vi "Main_Equip_1kw_ref742.vi"() -> ()   [LabVIEW 2025]
panel:
  out "hardware name":string
  out "isOnline 2":bool
  out "IndexSup":i32
  out "IndexInf":i32
  in  "Verifica":bool
  out "High Time":sgl format="%#_3g"
  out "Low Time":sgl format="%#_3g"
  in  "High Temp.":sgl
  in  "Low Temp.":sgl
  out "Temps":sgl caption="Time" format="%.1f"
  out "Calibration result:":bool
  out "error out_USB":errorcluster
  out "Nom Sensor Temperatura":string
  in  "Dades":sgl[](array[numeric])
  in  "Guardar 24h":bool caption="Informe"
  out "Dies":u8 caption="NumDies"
  in  "Reset_AutoSave 24":bool
  in  "mT1":sgl caption="Temperatura_1" format="%.1f"
  out "Maxim":sgl
  in  "BtSalir":bool caption="Sortir"
  in  "Reset_AutoSave":bool
  in  "Test name:":string
  out "Gràfiques T-Temps":cluster{"Value":sgl[], "Value":sgl[]}[](graph)
  in  "Datos OK":bool
  out "DadesComplertes":sgl[](array[numeric])
  in  "Grafica_OK":bool=TRUE
  out "Tabla":sgl[][](array[numeric])
  in  "Registro OK":bool=TRUE
  in  "time out":bool
  in  "Reset_gráfica":bool
  in  "Reset_Time":bool
  in  "Tiempo_string":string[](array[string])
  out "Elapsed Time (s)":i32
  out "Ensayo activo":bool
  out "FSenseTara":sgl caption="Fuerza - N"
  in  "CaptadorF":u16(ring) caption="Unidades" items=["25kg"=5]
  in  "PendentLlum":sgl caption="Força" format="%.1f"
  out "FactorsUnitatsPendents_F":dbl[](array[numeric])
  out "ConversioUnitatsF":dbl[](array[numeric])=[1.0, 9.8756, 2.2]
  out "ArraiUnitats":cluster{"String":string, "Value":u16}[](array[cluster])=[{"String"="kg", "Value"=0}, {"String"="N", "Value"=1}, {"String"="g", "Value"=2}, {"String"="daN", "Value"=3}, {"String"="cN", "Value"=4}, {"String"="KN", "Value"=5}, {"String"="lb", "Value"=6}]
  out "Tara":sgl caption="Força" format="%.1f"
  out "Temperatura1":sgl caption="Temperature" format="%.1f"
  out "PendentsT":sgl[](array[numeric])
  in  "Salir":bool caption="Sortir"
  in  "Ensayonuevo":bool caption="New Test"
  in  "Guardar":bool
  in  "Iniciar / Finalizar":bool=TRUE caption="Finalitzar prova"
  in  "UnidadesF":u16(ring) caption="Unidades" items=["kg", "N", "g"]
  in  "BtTaraPot":bool caption="TARA"
  # "sg"
  # "ºC"
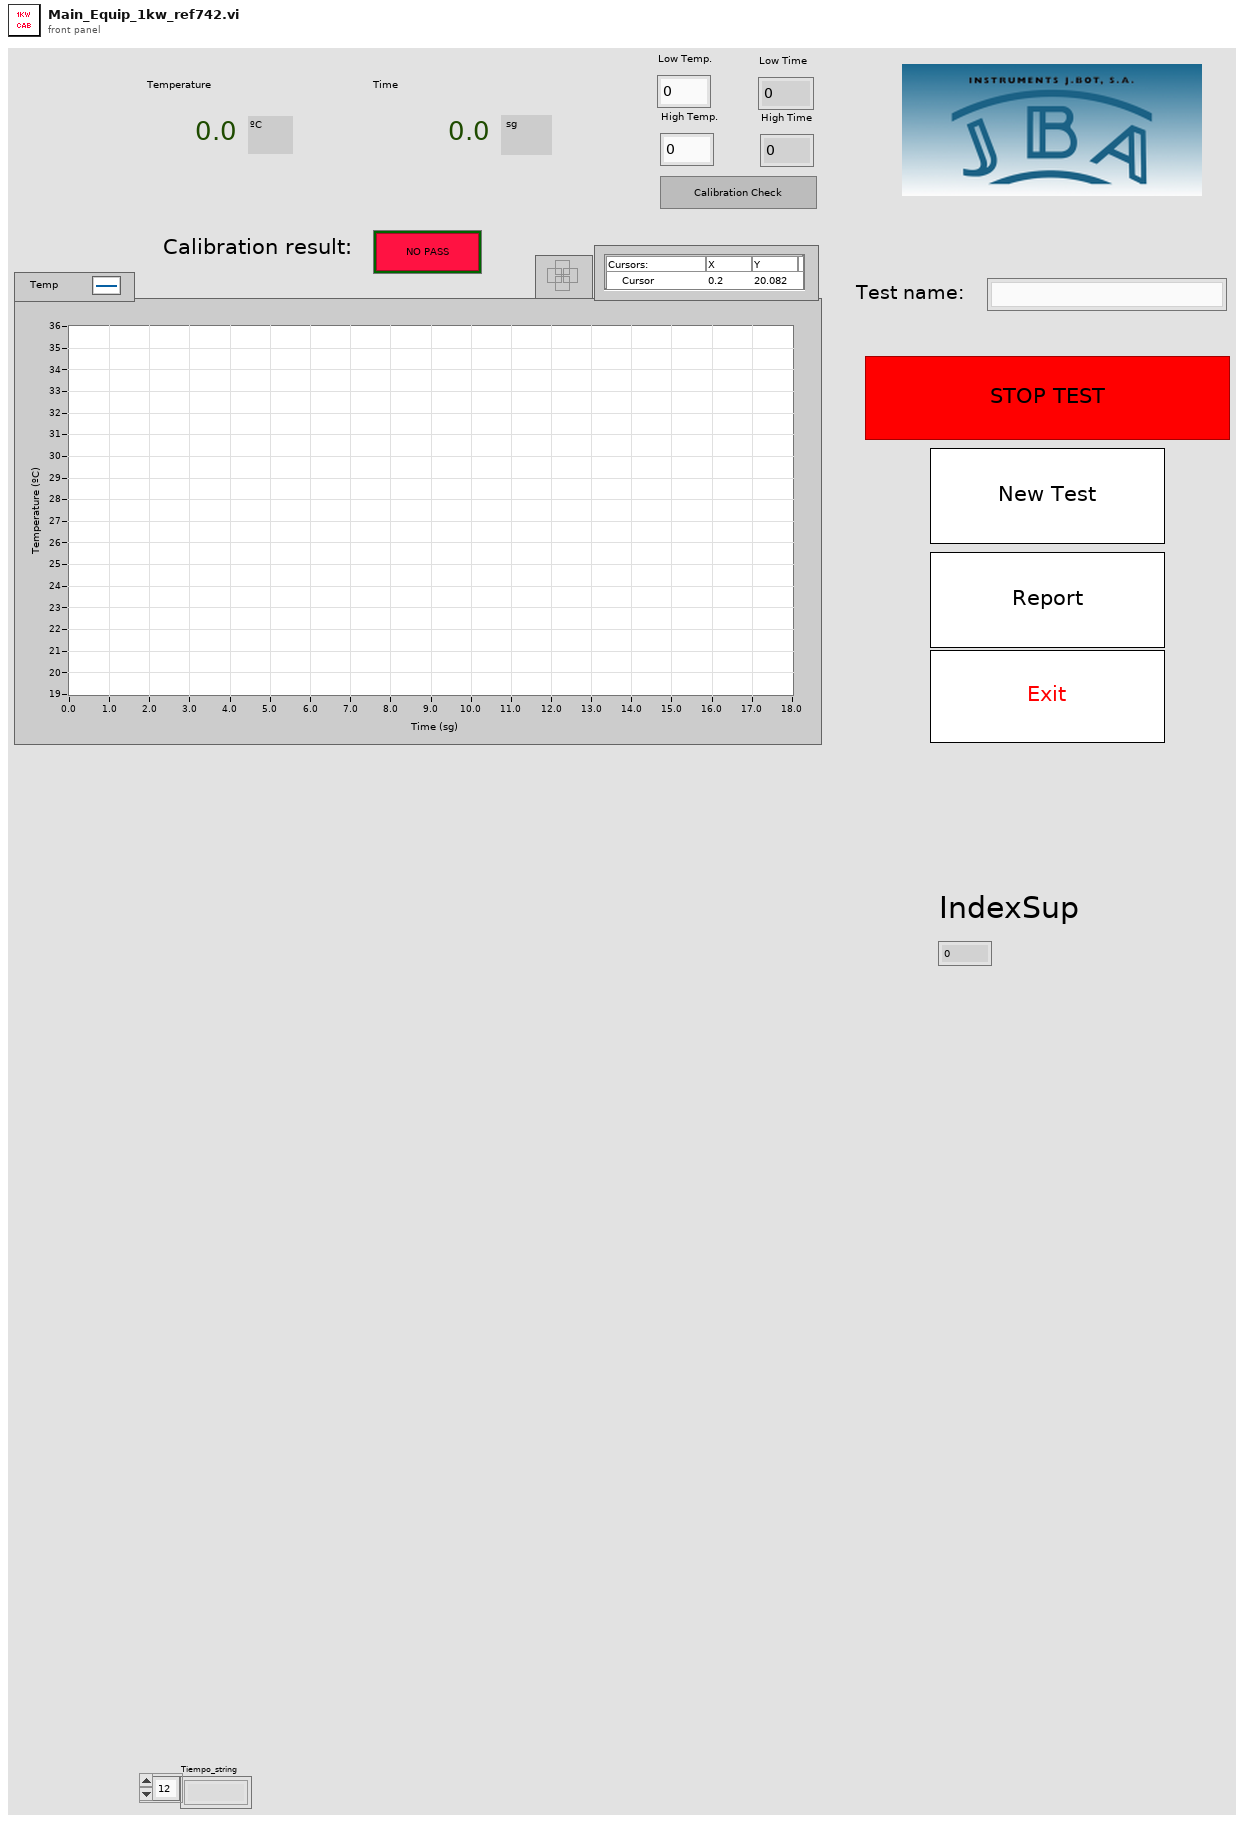
[diagram p1: front panel]
types:
  T1 = enum8{"Enabled", "Disabled", "Disabled and Grayed Out"}
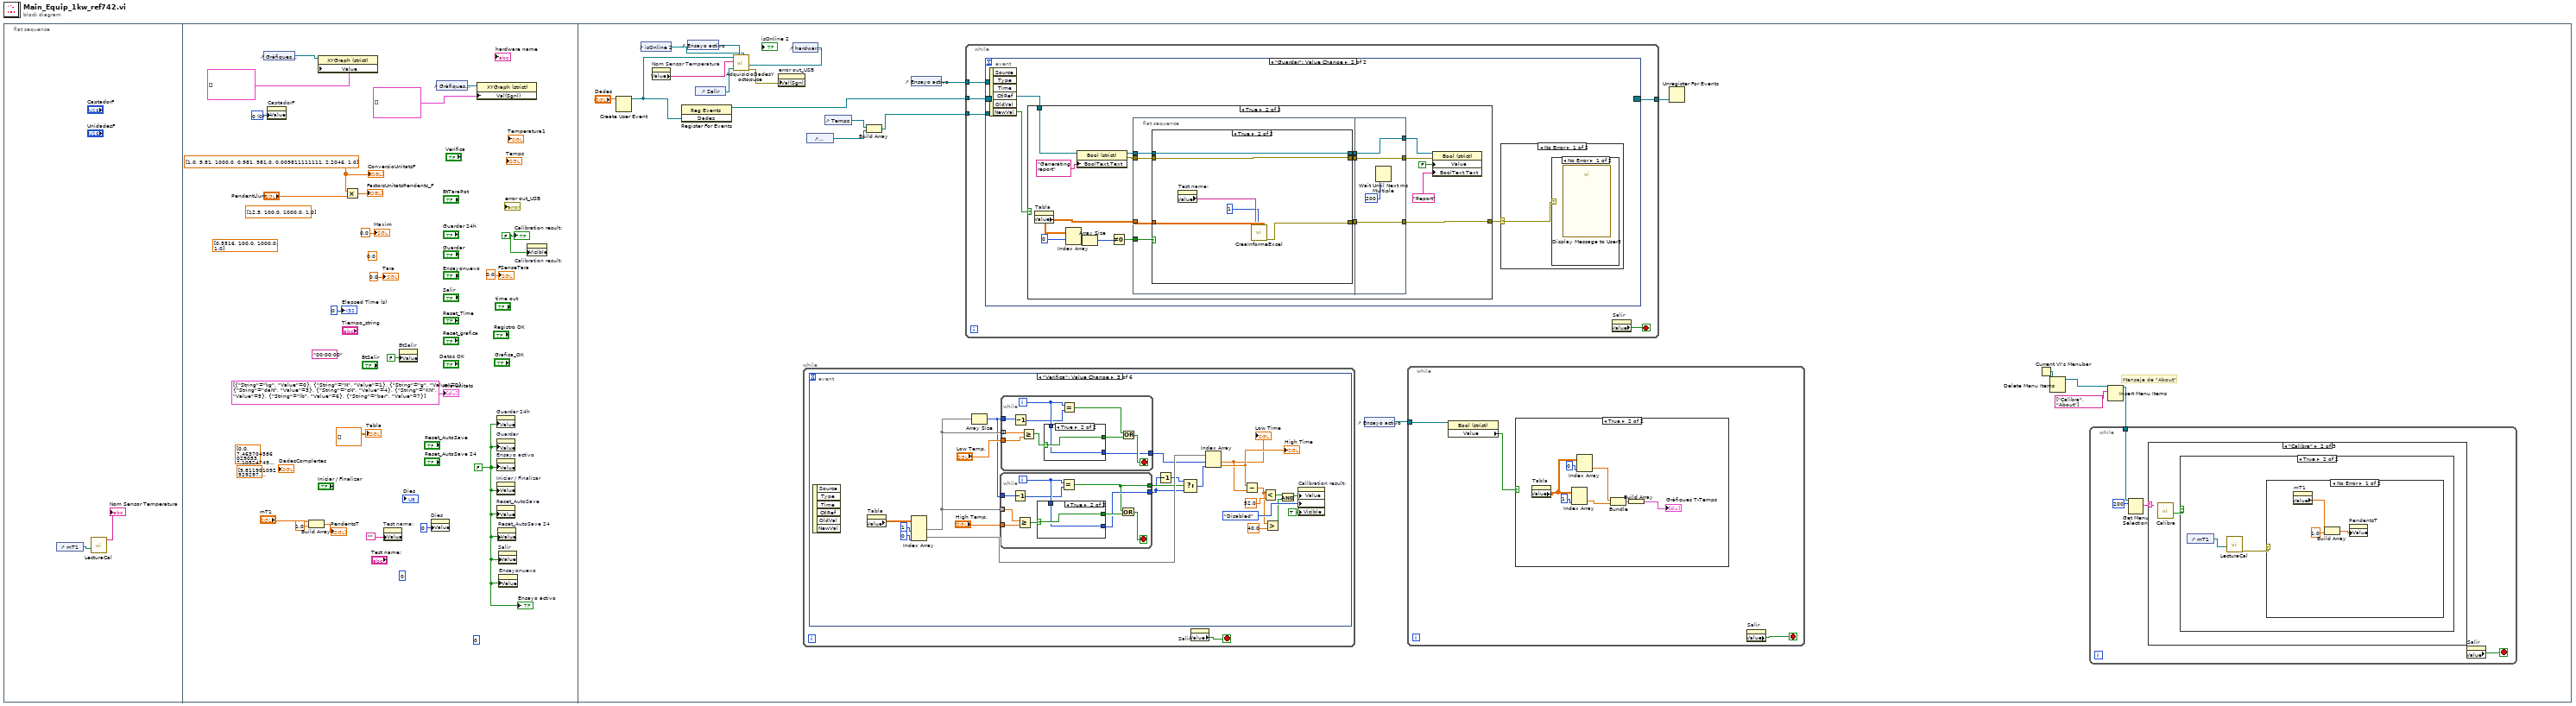
[diagram p0: block diagram]
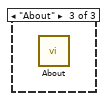
[diagram p5: hidden frame]
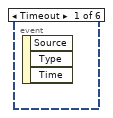
[diagram p7: hidden frame]
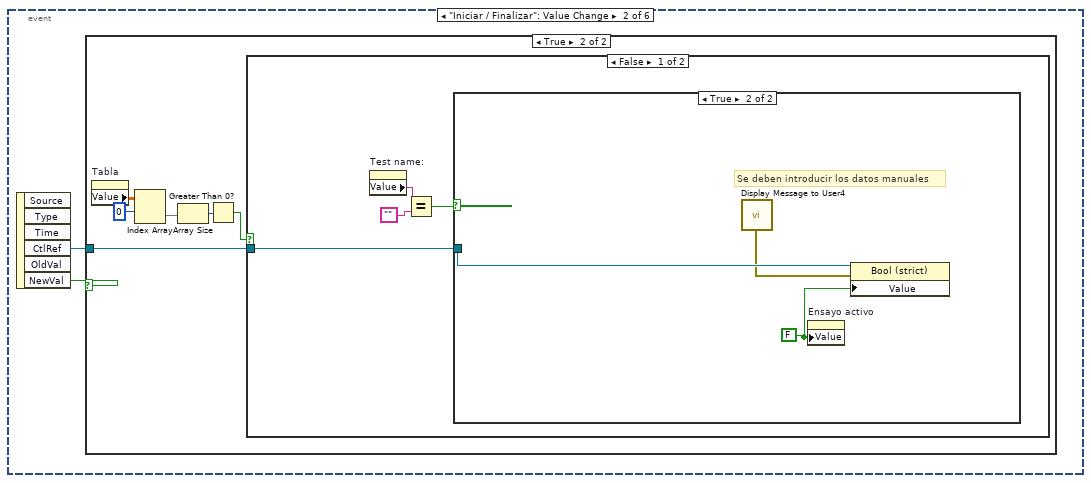
[diagram p8: hidden frame]
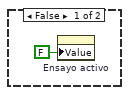
[diagram p9: hidden frame]
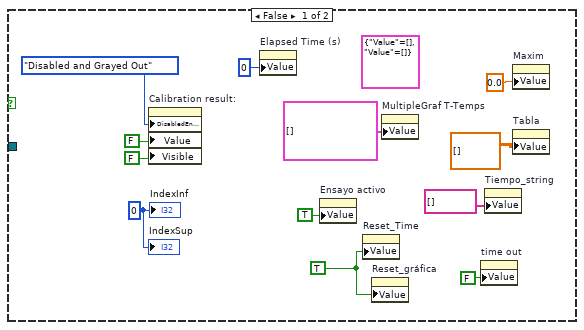
[diagram p10: hidden frame]
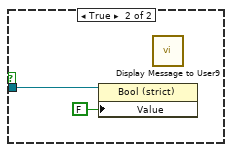
[diagram p11: hidden frame]
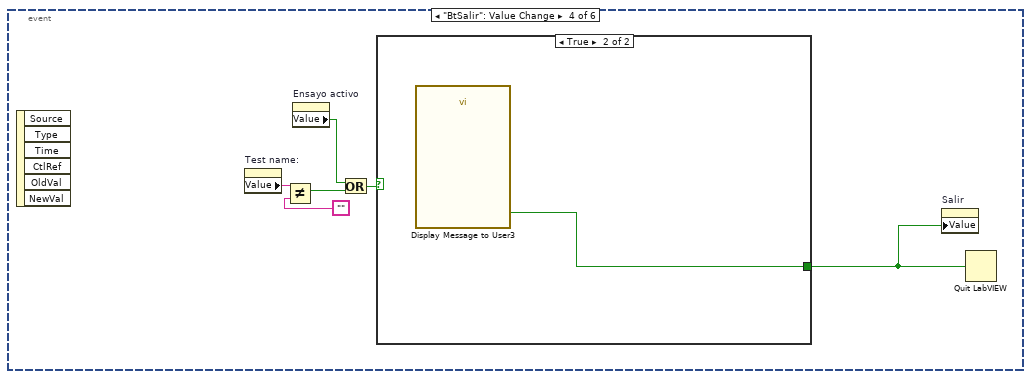
[diagram p14: hidden frame]
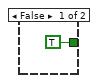
[diagram p15: hidden frame]
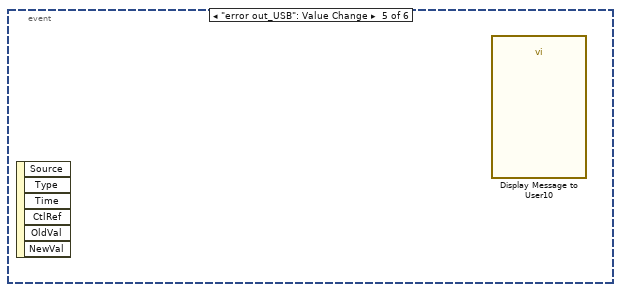
[diagram p16: hidden frame]
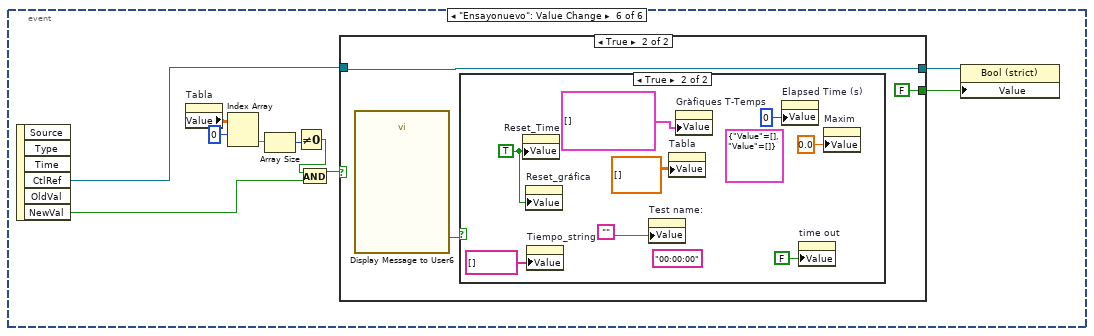
[diagram p17: hidden frame]
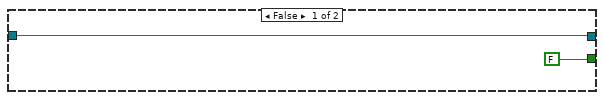
[diagram p18: hidden frame]
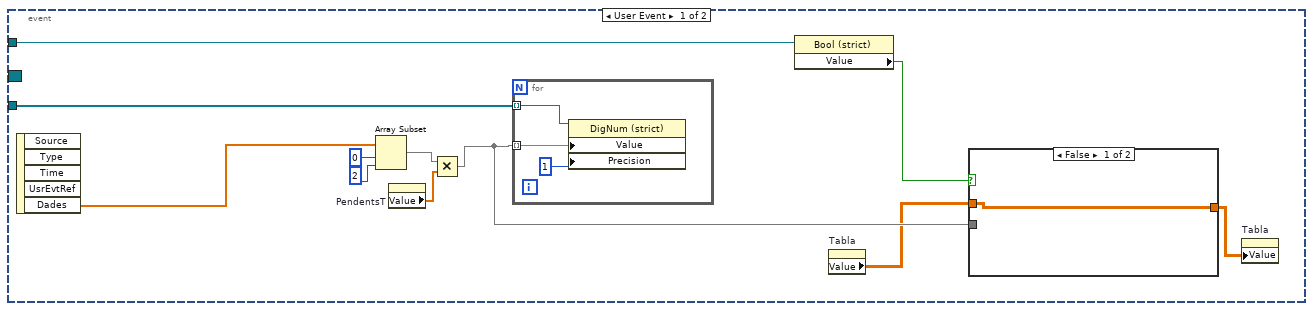
[diagram p20: hidden frame]
diagram:
  n1 = flat-sequence {
    frame #0 {
      n2 = control-ref of="mT1"() -> (w2:refnum<vi>)
      n3 = call "LecturaCal.vi"("T1"=w2) -> ("Nom Sensor Temperatura"=→"Nom Sensor Temperatura":string)  [unwired: 9 in, 1 out]
    }
    frame #1 {
      w3 = FALSE ("Resultat Assaig")
      (unwired) sgl[] [9.811901, 9.763803, 9.671529, 9.535354] ("DadesComplertes")
      (unwired) sgl[][] [[0.0, 7.4637046, 7.1052475, 6.7309566, 6.297442], [5.0, 2.5386999, 2.902987, 3.276568, 3.6958933], [10.0, 7.471229, 7.101099, 6.7181377, 6.2959595], [15.0, 2.5153666, 2.9171765, 3.291629, 3.679636], [20.0, 7.4759755, 7.089289, 6.711311, 6.298526]] ("Tabla")
      (unwired) u8 0 ("Durada assaig minuts")
      (unwired) u8 0 ("Durada assaig - hores:")
      w14 = u16 0 items=["0"] ("CaptadorF")
      (unwired) sgl 0.0 ("Fuerza")
      (unwired) dbl[] [0.5516, 100.0, 1000.0, 1.0] ("y")
      (unwired) "00:00:00" ("Tiempo transcurrido (hh:mm:ss)")
      w4 = FALSE ("Ensayo activo")
      (unwired) dbl[] [12.5, 100.0, 1000.0, 1.0] ("y")
      w23 = dbl[] [1.0, 9.81, 1000.0, 0.981, 981.0, 0.009811111111, 2.2046, 1.0]
      n4 = control-ref of="Gràfiques T-Temps"() -> (w6:refnum<vi>)
      n5 = property on="CaptadorF" class="Ring (strict)"("Value"=w14) -> ()  [unwired: 2 in, 2 out]
      n6 = Build Array("mT1", sgl 1.0 ("element")) -> (→"PendentsT":sgl[])
      n7 = property class="XYGraph (strict)"(reference=w6, "Value"=cluster{"Value":sgl[], "Value":sgl[]}[] []) -> ()  [unwired: 1 in, 2 out]
      n8 = Multiply(x=w23, y="PendentLlum") -> (x*y=→"FactorsUnitatsPendents_F":dbl[])
      n9 = property on="Test name:" class="Str"("Value"="") -> ()  [unwired: 2 in, 2 out]
      n10 = property on="BtSalir" class="Bool (strict)"("Value"=FALSE ("BtSalir")) -> ()  [unwired: 2 in, 2 out]
      n11 = property on="Dies" class="DigNum (strict)"("Value"=u8 0 ("NumDies")) -> ()  [unwired: 2 in, 2 out]
      n12 = control-ref of="Gràfiques T-Temps"() -> (w10:refnum<vi>)
      n13 = property class="XYGraph (strict)"(reference=w10, "Val(Sgnl)"=cluster{"Value":sgl[], "Value":sgl[]}[] [] ("Value")) -> ()  [unwired: 1 in, 2 out]
      n14 = property on="Guardar 24h" class="Bool (strict)"("Value"=w4) -> ()  [unwired: 2 in, 2 out]
      n15 = property on="Guardar" class="Bool (strict)"("Value"=w4) -> ()  [unwired: 2 in, 2 out]
      n16 = property on="Ensayo activo" class="Bool (strict)"("Value"=w4) -> ()  [unwired: 2 in, 2 out]
      n17 = property on="Iniciar / Finalizar" class="Bool (strict)"("Value"=w4) -> ()  [unwired: 2 in, 2 out]
      n18 = property on="Reset_AutoSave" class="Bool (strict)"("Value"=w4) -> ()  [unwired: 2 in, 2 out]
      n19 = property on="Reset_AutoSave 24" class="Bool (strict)"("Value"=w4) -> ()  [unwired: 2 in, 2 out]
      n20 = property on="Salir" class="Bool (strict)"("Value"=w4) -> ()  [unwired: 2 in, 2 out]
      n21 = property on="Ensayonuevo" class="Bool (strict)"("Value"=w4) -> ()  [unwired: 2 in, 2 out]
      n22 = property on="Calibration result:" class="Bool (strict)"("Visible"=w3) -> ()  [unwired: 2 in, 2 out]
      "Tara" <- sgl 0.0 ("Tara")
      "ArraiUnitats" <- cluster{"String":string, "Value":u16}[] [{"String"="kg", "Value"=0}, {"String"="N", "Value"=1}, {"String"="g", "Value"=2}, {"String"="daN", "Value"=3}, {"String"="cN", "Value"=4}, {"String"="KN", "Value"=5}, {"String"="lb", "Value"=6}, {"String"="bar", "Value"=7}] ("Strings And Values [] 2")
      "ConversioUnitatsF" <- w23
      "FSenseTara" <- sgl 0.0 ("FSenseTara")
      "Elapsed Time (s)" <- 0 ("Elapsed Time (s)")
      "Tabla" <- sgl[][] [] ("Tabla")
      "Maxim" <- sgl 0.0 ("Maxim")
      "Calibration result:" <- w3
      "Ensayo activo" <- w4
    }
    frame #2 {
      # "Mensaje de \"About\""
      n23 = Create User Event(user event datatype="Dades") -> (user event=w35:refnum<user-event>)  [unwired: 1 in, 1 out]
      n24 = control-ref of="isOnline 2"() -> (w26:refnum<vi>)
      n25 = property on="Nom Sensor Temperatura" class="Str"() -> ("Value"=w34:string)  [unwired: 2 in, 2 out]
      n26 = register-events(w35) -> (reference out=w42:refnum<event-registration>)  [unwired: 2 in, 1 out]
      n27 = control-ref of="Ensayo activo"() -> (w32:refnum<vi>)
      n28 = control-ref of="Salir"() -> (w41:refnum<vi>)
      n29 = control-ref of="hardware name"() -> (w25:refnum<vi>)
      n30 = call "AdquisicioDadesYoctopuce.vi"("HardName"=w25, "online?"=w26, "AssaigActiu"=w32, "Stop"=w41, "Temperature name"=w34, "user event in"=w35) -> ("error out"=w33:errorcluster)  [unwired: 4 in, 1 out]
      n31 = property on="error out_USB" class="Clust (strict)"("Val(Sgnl)"=w33) -> ()  [unwired: 2 in, 2 out]
      n32 = while {
        stop <- w64 stop-if-true
        n33 = event shown="[2] \"Verifica\": Value Change" {
          selector: _ -> [_ _ _ _ _ _]
          dyn-events: _ -> [_ _ _ _ _ _]
          timeout: _ -> [_ _ _ _ _ _]
          event Timeout {
            n34 = event-data() -> ()  [unwired: 1 in, 3 out]
          }
          event "Iniciar / Finalizar": Value Change {
            n35 = event-data() -> ("CtlRef"=w65:refnum<vi>, "NewVal"=w66:bool)  [unwired: 1 in, 4 out]
            n36 = case shown="True" w66 {
              tunnel: w65 -> [_ w73]
              frame False {
                n37 = property on="Ensayo activo" class="Bool (strict)"("Value"=FALSE ("Ensayo activo")) -> ()  [unwired: 2 in, 2 out]
              }
              frame True {
                n38 = property on="Tabla" class="Arr (strict)"() -> ("Value"=w72:sgl[][])  [unwired: 2 in, 2 out]
                n39 = Index Array(array=w72, index (row)=0) -> (element=w71:sgl[])  [unwired: 1 in]
                n40 = Array Size(array=w71) -> (size(s)=w69:i32)
                n41 = Greater Than 0?(x=w69) -> (x > 0?=w68:bool)
                n42 = case shown="False" w68 {
                  tunnel: w73 -> [w77 w94]
                  frame False {
                    n43 = property on="Test name:" class="Str"() -> ("Value"=w76:string)  [unwired: 2 in, 2 out]
                    n44 = Equal?(x=w76, y="") -> (x = y?=w74:bool)
                    n45 = case shown="True" w74 {
                      tunnel: w77 -> [_ w92]
                      frame False {
                        w78 = 0 ("IndexInf")
                        (unwired) cluster{"Value":sgl[], "Value":sgl[]} {"Value"=[], "Value"=[]} ("Grafica F-T")
                        w87 = TRUE ("Reset_Time")
                        n46 = property on="Calibration result:" class="Bool (strict)"("DisabledEnum"=T1."Disabled and Grayed Out" ("Disabled"), "Value"=FALSE ("Resultat Assaig"), "Visible"=FALSE) -> ()  [unwired: 2 in, 2 out]
                        n47 = property on="Elapsed Time (s)" class="DigNum (strict)"("Value"=0 ("Elapsed Time (s)")) -> ()  [unwired: 2 in, 2 out]
                        n48 = property on="Ensayo activo" class="Bool (strict)"("Value"=TRUE ("Iniciar assaig")) -> ()  [unwired: 2 in, 2 out]
                        n49 = property on="Reset_Time" class="Bool (strict)"("Value"=w87) -> ()  [unwired: 2 in, 2 out]
                        n50 = property on="Reset_gráfica" class="Bool (strict)"("Value"=w87) -> ()  [unwired: 2 in, 2 out]
                        n51 = property on="MultipleGraf T-Temps" class="XYGraph (strict)"("Value"=cluster{"Y":dbl[], "Y":dbl[]}[] []) -> ()  [unwired: 2 in, 2 out]
                        n52 = property on="time out" class="Bool (strict)"("Value"=FALSE ("time out")) -> ()  [unwired: 2 in, 2 out]
                        n53 = property on="Tiempo_string" class="Arr (strict)"("Value"=string[] [] ("Tiempo_string")) -> ()  [unwired: 2 in, 2 out]
                        n54 = property on="Maxim" class="DigNum (strict)"("Value"=sgl 0.0 ("Maxim")) -> ()  [unwired: 2 in, 2 out]
                        n55 = property on="Tabla" class="Arr (strict)"("Value"=sgl[][] [] ("Tabla")) -> ()  [unwired: 2 in, 2 out]
                        "IndexSup" <- w78
                        "IndexInf" <- w78
                      }
                      frame True {
                        w91 = FALSE
                        # "Se deben introducir los datos manuales"
                        n56 = call "Display Message to User4"() -> ("error out"=w90:errorcluster)  [unwired: 10 in, 1 out]
                        n57 = property on="Ensayo activo" class="Bool (strict)"("Value"=w91) -> ()  [unwired: 2 in, 2 out]
                        n58 = property class="Bool (strict)"(reference=w92, error in=w90, "Value"=w91) -> ()  [unwired: 2 out]
                      }
                    }
                  }
                  frame True {
                    n59 = property class="Bool (strict)"(reference=w94, "Value"=FALSE) -> ()  [unwired: 1 in, 2 out]
                    n60 = call "Display Message to User9"() -> ()  [unwired: 10 in, 2 out]
                  }
                }
              }
            }
          }
          event "Verifica": Value Change {
            n61 = event-data() -> ()  [unwired: 1 in, 6 out]
            n62 = property on="Tabla" class="Arr (strict)"() -> ("Value"=w117:sgl[][])  [unwired: 2 in, 2 out]
            n63 = Index Array(array=w117, index (col) #1=1 ("index (row)"), index (col) #2=0 ("index (row)")) -> (element #1=w108:sgl[], element #2=w105:sgl[])  [unwired: 2 in]
            n64 = Array Size(array=w108) -> (size(s)=w106:i32)
            n65 = while {
              tunnel: w108 -> [w127] mode=indexing
              tunnel: "High Temp." -> [w121]
              tunnel: w106 -> [w120]
              tunnel: [w119] -> w95
              tunnel: [w118] -> w98
              i -> [w125]
              stop <- w122 stop-if-true
              n66 = Decrement(x=w120) -> (x-1=w124:i32)
              n67 = Greater Or Equal?(x=w127, y=w121) -> (x >= y?=w126:bool)
              n68 = case shown="True" w126 {
                selector: w126 -> [w128 w130]
                tunnel: w125 -> [_ w129]
                tunnel: [w128 w130] -> w123
                tunnel: [_ w129] -> w119
                frame False {
                }
                frame True {
                }
              }
              n69 = Equal?(x=w125, y=w124) -> (x = y?=w118:bool)
              n70 = Or(x=w118, y=w123) -> (x .or. y?=w122:bool)
            }
            n71 = while {
              tunnel: w108 -> [w140] mode=indexing
              tunnel: "Low Temp." -> [w139]
              tunnel: w106 -> [w136]
              tunnel: [w131] -> w104
              i -> [w137]
              stop <- w132 stop-if-true
              n72 = Decrement(x=w136) -> (x-1=w135:i32)
              n73 = Greater Or Equal?(x=w140, y=w139) -> (x >= y?=w138:bool)
              n74 = case shown="True" w138 {
                selector: w138 -> [w141 w143]
                tunnel: w137 -> [_ w142]
                tunnel: [w141 w143] -> w133
                tunnel: [_ w142] -> w131
                frame False {
                }
                frame True {
                }
              }
              n75 = Equal?(x=w137, y=w135) -> (x = y?=w134:bool)
              n76 = Or(x=w134, y=w133) -> (x .or. y?=w132:bool)
            }
            n77 = Decrement(x=w95) -> (x-1=w96:i32)
            n78 = Select(t=w96, s=w98, f=w95) -> (s? t:f=w97:i32)
            n79 = Index Array(array=w105, index #1=w104, index #2=w97) -> (element #1=w112:sgl, element #2=w113:sgl)
            "Low Time" <- w112
            "High Time" <- w113
            n80 = Subtract(x=w113, y=w112) -> (x-y=w102:sgl)
            n81 = Less?(x=w102, y=sgl 52.0) -> (x < y?=w100:bool)
            n82 = Greater?(x=w102, y=40.0) -> (0:w99:bool)
            n83 = And(x=w100, y=w99) -> (x .and. y?=w101:bool)
            n84 = property on="Calibration result:" class="Bool (strict)"("Value"=w101, "DisabledEnum"=T1."Disabled" ("Disabled"), "Visible"=TRUE) -> ()  [unwired: 2 in, 2 out]
          }
          event "BtSalir": Value Change {
            n85 = event-data() -> ()  [unwired: 1 in, 6 out]
            n86 = property on="Test name:" class="Str"() -> ("Value"=w148:string)  [unwired: 2 in, 2 out]
            n87 = Not Equal?(x=w148, y="") -> (x != y?=w144:bool)
            n88 = property on="Ensayo activo" class="Bool (strict)"() -> ("Value"=w145:bool)  [unwired: 2 in, 2 out]
            n89 = Or(x=w145, y=w144) -> (x .or. y?=w146:bool)
            n90 = case shown="True" w146 {
              tunnel: [TRUE ("OK") w151] -> w149
              frame False {
              }
              frame True {
                n91 = call "Display Message to User3"() -> ("OK"=w151:bool)  [unwired: 10 in, 1 out]
              }
            }
            n92 = property on="Salir" class="Bool (strict)"("Value"=w149) -> ()  [unwired: 2 in, 2 out]
            n93 = Quit LabVIEW(quit? (T)=w149) -> ()
          }
          event "error out_USB": Value Change {
            n94 = event-data() -> ()  [unwired: 1 in, 6 out]
            n95 = call "Display Message to User10"() -> ()  [unwired: 10 in, 2 out]
          }
          event "Ensayonuevo": Value Change {
            n96 = event-data() -> ("CtlRef"=w159:refnum<vi>, "NewVal"=w152:bool)  [unwired: 1 in, 4 out]
            n97 = property on="Tabla" class="Arr (strict)"() -> ("Value"=w157:sgl[][])  [unwired: 2 in, 2 out]
            n98 = Index Array(array=w157, index (row)=0) -> (element=w154:sgl[])  [unwired: 1 in]
            n99 = Array Size(array=w154) -> (size(s)=w155:i32)
            n100 = Not Equal To 0?(x=w155) -> (x != 0?=w153:bool)
            n101 = And(x=w153, y=w152) -> (x .and. y?=w158:bool)
            n102 = case shown="True" w158 {
              tunnel: w159 -> [w163 w165]
              tunnel: [w163 w165] -> w160
              tunnel: [FALSE ("Value") FALSE ("Value")] -> w161
              frame False {
              }
              frame True {
                n103 = call "Display Message to User6"() -> ("Yes"=w166:bool)  [unwired: 10 in, 1 out]
                n104 = case shown="True" w166 {
                  frame False {
                  }
                  frame True {
                    (unwired) "00:00:00" ("Tiempo transcurrido (hh:mm:ss)")
                    w171 = TRUE ("Reset_Time")
                    (unwired) cluster{"Value":sgl[], "Value":sgl[]} {"Value"=[], "Value"=[]} ("Grafica F-T")
                    n105 = property on="Reset_Time" class="Bool (strict)"("Value"=w171) -> ()  [unwired: 2 in, 2 out]
                    n106 = property on="Reset_gráfica" class="Bool (strict)"("Value"=w171) -> ()  [unwired: 2 in, 2 out]
                    n107 = property on="Tiempo_string" class="Arr (strict)"("Value"=string[] [] ("Tiempo_string")) -> ()  [unwired: 2 in, 2 out]
                    n108 = property on="Test name:" class="Str"("Value"="") -> ()  [unwired: 2 in, 2 out]
                    n109 = property on="Tabla" class="Arr (strict)"("Value"=sgl[][] [] ("Tabla")) -> ()  [unwired: 2 in, 2 out]
                    n110 = property on="Gràfiques T-Temps" class="XYGraph (strict)"("Value"=cluster{"Y":dbl[], "Y":dbl[]}[] []) -> ()  [unwired: 2 in, 2 out]
                    n111 = property on="Elapsed Time (s)" class="DigNum (strict)"("Value"=0 ("Elapsed Time (s)")) -> ()  [unwired: 2 in, 2 out]
                    n112 = property on="time out" class="Bool (strict)"("Value"=FALSE ("time out")) -> ()  [unwired: 2 in, 2 out]
                    n113 = property on="Maxim" class="DigNum (strict)"("Value"=sgl 0.0 ("Maxim")) -> ()  [unwired: 2 in, 2 out]
                  }
                }
              }
            }
            n114 = property class="Bool (strict)"(reference=w160, "Value"=w161) -> ()  [unwired: 1 in, 2 out]
          }
        }
        n115 = property on="Salir" class="Bool (strict)"() -> ("Value"=w64:bool)  [unwired: 2 in, 2 out]
      }
      n116 = control-ref of="Temperatura1"() -> (w27:refnum<vi>)
      n117 = control-ref of="Temps"() -> (w28:refnum<vi>)
      n118 = Build Array(w28, w27) -> (w31:refnum<vi>[])
      n119 = control-ref of="Ensayo activo"() -> (w30:refnum<vi>)
      n120 = while {
        tunnel: w42 -> [w179]
        tunnel: [w178] -> w43
        tunnel: w31 -> [w176]
        tunnel: w30 -> [w175]
        stop <- w177 stop-if-true
        n121 = event shown="[1] \"Guardar\": Value Change" {
          selector: w179 -> [_ _]
          dyn-events: [_ _] -> w178
          timeout: _ -> [_ _]
          tunnel: w176 -> [w185 _]
          tunnel: w175 -> [w184 _]
          event User Event {
            n122 = event-data() -> ("Dades"=w187:sgl[])  [unwired: 1 in, 4 out]
            n123 = Array Subset(array=w187, index=0, length=2) -> (w188:sgl[])
            n124 = property on="PendentsT" class="Arr (strict)"() -> ("Value"=w186:sgl[])  [unwired: 2 in, 2 out]
            n125 = Multiply(x=w188, y=w186) -> (x*y=w182:sgl[])
            n126 = for {
              tunnel: w185 -> [w191] mode=indexing
              tunnel: w182 -> [w192] mode=indexing
              n127 = property class="DigNum (strict)"(reference=w191, "Value"=w192, "Precision"=u8 1 ("Display Format:Precision")) -> ()  [unwired: 1 in, 2 out]
            }
            n128 = property class="Bool (strict)"(reference=w184) -> ("Value"=w183:bool)  [unwired: 1 in, 2 out]
            n129 = property on="Tabla" class="Arr (strict)"() -> ("Value"=w181:sgl[][])  [unwired: 2 in, 2 out]
            n130 = case shown="False" w183 {
              tunnel: w182 -> [_ w197]
              tunnel: w181 -> [w194 w196]
              tunnel: [w194 w195] -> w180
              frame False {
              }
              frame True {
                n131 = Build Array (concatenate)(w196, w197) -> (w195:sgl[][])
              }
            }
            n132 = property on="Tabla" class="Arr (strict)"("Value"=w180) -> ()  [unwired: 2 in, 2 out]
          }
          event "Guardar": Value Change {
            n133 = event-data() -> ("CtlRef"=w198:refnum<vi>, "NewVal"=w200:bool)  [unwired: 1 in, 4 out]
            n134 = case shown="True" w200 {
              tunnel: [errorcluster {"status"=FALSE, "code"=0, "source"=""} ("error out") w220] -> w199
              tunnel: w198 -> [_ w210]
              frame False {
              }
              frame True {
                n135 = property on="Tabla" class="Arr (strict)"() -> ("Value"=w204:sgl[][])  [unwired: 2 in, 2 out]
                n136 = Index Array(array=w204, index (row)=0) -> (element=w218:sgl[])  [unwired: 1 in]
                n137 = property class="Bool (strict)"(reference=w210, "BoolText.Text"="Generating report" ("Boolean Text.Text")) -> (reference out=w209:refnum<vi>, error out=w205:errorcluster)  [unwired: 1 in]
                n138 = Array Size(array=w218) -> (size(s)=w206:i32)
                n139 = Not Equal To 0?(x=w206) -> (x != 0?=w217:bool)
                n140 = flat-sequence {
                  tunnel: w204 -> [w226]
                  tunnel: w217 -> [w225]
                  tunnel: w209 -> [w223]
                  tunnel: [w227] -> w213
                  tunnel: [w224] -> w212
                  tunnel: [w222] -> w211
                  tunnel: w205 -> [w221]
                  tunnel: [w238] -> w215
                  tunnel: [w239] -> w216
                  tunnel: [w240] -> w220
                  tunnel: w213 -> [w240]
                  tunnel: w212 -> [w239]
                  tunnel: w211 -> [w238]
                  frame #0 {
                    n141 = case shown="True" w225 {
                      tunnel: [errorcluster {"status"=TRUE, "code"=0, "source"=""} ("error out") w233] -> w227
                      tunnel: w226 -> [_ w235]
                      tunnel: [w229 w232] -> w224
                      tunnel: w223 -> [w228 w236]
                      tunnel: [w228 w236] -> w222
                      tunnel: w221 -> [_ w232]
                      frame False {
                        n142 = call "Display Message to User8"() -> ("error out"=w229:errorcluster)  [unwired: 10 in, 1 out]
                      }
                      frame True {
                        n143 = property on="Test name:" class="Str"() -> ("Value"=w234:string)  [unwired: 2 in, 2 out]
                        n144 = call "CreaInformeExcel.vi"("Nom Assaig"=w234, "NºTests"=u8 1, "Tabla"=w235) -> ("error out"=w233:errorcluster)  [unwired: 15 in, 1 out]
                      }
                    }
                  }
                  frame #1 {
                    n145 = Wait Until Next ms Multiple(millisecond multiple=u32 200 ("milliseconds to wait")) -> ()  [unwired: 1 out]
                  }
                }
                n146 = property class="Bool (strict)"(reference=w215, error in=w216, "Value"=FALSE, "BoolText.Text"="Report" ("Boolean Text.Text")) -> ()  [unwired: 2 out]
              }
            }
            n147 = case shown="No Error" w199 {
              selector: w199 -> [w201 _]
              frame No Error {
                n148 = case shown="No Error" w201 {
                  frame No Error {
                    n149 = call "Display Message to User5"() -> ()  [unwired: 10 in, 2 out]
                  }
                  frame Error {
                    n150 = property on="Reset_AutoSave" class="Bool (strict)"("Value"=FALSE ("Reset_AutoSave")) -> ()  [unwired: 2 in, 2 out]
                  }
                }
              }
              frame Error {
              }
            }
          }
        }
        n151 = property on="Salir" class="Bool (strict)"() -> ("Value"=w177:bool)  [unwired: 2 in, 2 out]
      }
      n152 = control-ref of="Ensayo activo"() -> (w29:refnum<vi>)
      n153 = while {
        tunnel: w29 -> [w55]
        stop <- w56 stop-if-true
        n154 = property class="Bool (strict)"(reference=w55) -> ("Value"=w54:bool)  [unwired: 1 in, 2 out]
        n155 = case shown="True" w54 {
          frame False {
          }
          frame True {
            n156 = property on="Tabla" class="Arr (strict)"() -> ("Value"=w59:sgl[][])  [unwired: 2 in, 2 out]
            n157 = Index Array(array=w59, index (col)=1 ("index")) -> (element=w58:sgl[])  [unwired: 1 in]
            n158 = Index Array(array=w59, index (col)=0 ("index (row)")) -> (element=w57:sgl[])  [unwired: 1 in]
            n159 = Bundle("Value"=w57, "Value"=w58) -> (w63:cluster{"Value":sgl[], "Value":sgl[]})  [unwired: 1 in]
            n160 = Build Array(w63) -> (→"Gràfiques T-Temps":cluster{"Value":sgl[], "Value":sgl[]}[])
          }
        }
        n161 = property on="Salir" class="Bool (strict)"() -> ("Value"=w56:bool)  [unwired: 2 in, 2 out]
      }
      n162 = Unregister For Events(event registration refnum=w43) -> ()  [unwired: 1 in, 1 out]
      n163 = Current VI's Menubar() -> (w40:refnum<k9>)
      n164 = Delete Menu Items(9:w40) -> (3:w39:refnum<k9>)  [unwired: 3 in, 1 out]
      n165 = Insert Menu Items(8:string[] ["Calibra", "About"] ("item names"), 9:w39) -> (3:w38:refnum<k9>)  [unwired: 4 in, 2 out]
      n166 = while {
        tunnel: w38 -> [w45]
        stop <- w47 stop-if-true
        n167 = Get Menu Selection(0:w45, 1:200 ("ms timeout (200)")) -> (6:w44:string)  [unwired: 2 in, 4 out]
        n168 = case shown="\"Calibra\"" w44 {
          frame "False", Default {
          }
          frame "Calibra" {
            n169 = call "Calibra.vi"() -> ("SurtOk?"=w48:bool)  [unwired: 11 in]
            n170 = case shown="True" w48 {
              frame False {
              }
              frame True {
                n171 = control-ref of="mT1"() -> (w50:refnum<vi>)
                n172 = call "LecturaCal.vi"("T1"=w50) -> ("error out"=w49:errorcluster)  [unwired: 9 in, 1 out]
                n173 = case shown="No Error" w49 {
                  frame No Error {
                    n174 = property on="mT1" class="DigNum (strict)"() -> ("Value"=w53:sgl)  [unwired: 2 in, 2 out]
                    n175 = Build Array(w53, sgl 1.0 ("element")) -> (w52:sgl[])
                    n176 = property on="PendentsT" class="Arr (strict)"("Value"=w52) -> ()  [unwired: 2 in, 2 out]
                  }
                  frame Error {
                  }
                }
              }
            }
          }
          frame "About" {
            n177 = call "About.vi"() -> ()  [unwired: 1 in]
          }
        }
        n178 = property on="Salir" class="Bool (strict)"() -> ("Value"=w47:bool)  [unwired: 2 in, 2 out]
      }
    }
  }
